vi "find_handle_pose.vi"(7 "Parameters":T1={"Stimulus"={"Type"=enum."Off", "Delay"=0, "Amplitude"=[0.0, 0.0, 0.0], "Injection point"=enum."Total pose", "Closed loop"=FALSE, "Offset"=[0.0, 0.0, 0.0], "Tip -> world"=TRUE}, "Goal Filter A"={"Lower Fc"=0.0, "Lower Q"=0.15, "Scale factor"=0.0, "Upper Fc"=0.0075, "Upper Q"=0.01, "Manip zeroing"=0.001, "Speedup max"=150.0, "Speedup thresh"=5.0, "Speedup nonlin"=3.0, "V limit"=300.0, "V limit range"=300.0}, "Mode controls"={"Hold"=FALSE, "Cancellation"=FALSE, "Goal filter"=FALSE, "Trigger"=FALSE}, "Manipulator type"=enum."Current piezo", "Manipulator calibration"={"Inverse Kinematics"=[[-0.4736411481566654, -0.25724305819165183, -1.1087933259307599], [0.296735958809338, -0.258643951607561, -1.0971603505753995], [-0.043664688535758014, 0.44635679599468125, -1.1035515399424176]], "Handle transform"=[[3.281333089700394, 0.23462731743748497, 0.17832137948371765, -8265.081657965618], [-0.20249098046098263, 2.6933210343964133, -0.2815002765708058, -33565.66155248382], [-0.14581170473284072, 0.6821648518522063, 0.8833544952169589, 26862.18782130476], [-1.1202010727438122e-18, 5.861467994999758e-19, 1.760134464394436e-18, 0.999999999999992]], "Tip offset"=[0.0, 0.0, 36200.0], "Probe calibration"=[], "Pivot position"=[0.0, 0.0, -11360.0], "Axial filter"={"filter structure"=enum."IIR 2nd Order", "Reverse Coefficients"=[0.0, 0.0], "Forward Coefficients"=[1.0, 0.0, 0.0]}, "Lateral filter"={"filter structure"=enum."IIR 2nd Order", "Reverse Coefficients"=[0.0, 0.0], "Forward Coefficients"=[1.0, 0.0, 0.0]}}, "Charge piezo"={"Capacitance"=4e-08, "V min"=-235.0, "V max"=50.0, "- margin"=465.0, "+ margin"=0.001, "I max"=40000.0, "I sat"=90000000.0, "R series"=5.0, "R shunt"=1000.0, "Fault V"=0.0, "Start Fault V"=0.0, "Start Cycles"=0, "Prop gain"=1e-06, "Int gain"=0.0, "Diff gain"=0.0}, "Network"={"Remote Host"="192.168.1.3", "Send Status"=TRUE, "Send Port"=0, "Recv Commands"=FALSE, "Recv Port"=0}, "Goal Filter B"={"Lower Fc"=1.0, "Lower Q"=2.0, "Scale factor"=61557.0, "Upper Fc"=20.0, "Upper Q"=61557.0, "Manip zeroing"=2.0, "Speedup max"=1.0, "Speedup thresh"=300.0, "Speedup nonlin"=3.0, "V limit"=300.0, "V limit range"=300.0}, "Cancellation"={"Bandwidth"=0.0, "Delay"=0, "Stack travel"=0.0, "Saturation pos"=0.0075, "Slew Limit"=0.01, "Turnoff zeroing"=0.001, "Bypass"=FALSE}, "Transition time"=3.0} {"Transition time" format="%_3f"; "Cancellation"."Slew Limit" format="%#_3p"; "Cancellation"."Saturation pos" format="%#.1f"; "Cancellation"."Stack travel" format="%#.1f"; "Cancellation"."Turnoff zeroing" format="%#_6e"; "Cancellation"."Delay" step=1; "Cancellation"."Bandwidth" min=10 max=1000 step=10; "Goal Filter B"."V limit range" format="%_3p"; "Goal Filter B"."V limit" format="%_3p"; "Goal Filter B"."Speedup nonlin" format="%_3p"; "Goal Filter B"."Upper Q" format="%_3f"; "Goal Filter B"."Upper Fc" format="%_3p"; "Goal Filter B"."Lower Q" format="%_3f"; "Goal Filter B"."Speedup thresh" format="%_3p"; "Goal Filter B"."Speedup max" format="%_3p"; "Goal Filter B"."Manip zeroing" format="%_3p"; "Goal Filter B"."Scale factor" format="%_3f"; "Goal Filter B"."Lower Fc" format="%_3p"; "Charge piezo"."I sat" format="%#_6p"; "Charge piezo"."+ margin" format="%#_6p"; "Charge piezo"."- margin" format="%#_6p"; "Charge piezo"."Start Fault V" format="%#_6p"; "Charge piezo"."R shunt" format="%#_6p"; "Charge piezo"."Prop gain" format="%#_6p"; "Charge piezo"."Fault V" format="%#_6p"; "Charge piezo"."I max" format="%#_6p"; "Charge piezo"."Diff gain" format="%#_6p"; "Charge piezo"."Int gain" format="%#_6p"; "Charge piezo"."R series" format="%#_6p"; "Charge piezo"."Capacitance" format="%#_6p"; "Manipulator calibration"."Probe calibration" format="%#.1f"; "Manipulator calibration"."Handle transform" format="%#_3f"; "Manipulator calibration"."Inverse Kinematics" format="%#_3f"; "Goal Filter A"."V limit range" format="%_3p"; "Goal Filter A"."V limit" format="%_3p"; "Goal Filter A"."Speedup nonlin" format="%_3p"; "Goal Filter A"."Upper Q" format="%_3f"; "Goal Filter A"."Upper Fc" format="%_3p"; "Goal Filter A"."Lower Q" format="%_3f"; "Goal Filter A"."Speedup thresh" format="%_3p"; "Goal Filter A"."Speedup max" format="%_3p"; "Goal Filter A"."Manip zeroing" format="%_3p"; "Goal Filter A"."Scale factor" format="%_3f"; "Goal Filter A"."Lower Fc" format="%_3p"; "Stimulus"."Offset" step=100; "Stimulus"."Amplitude" step=100; "Stimulus"."Delay" step=100}, 10 "Zeroing offset":sgl[](array[numeric])) -> (0 "Handle pose":T7 format="%#_5f", 1 "Central tip position":sgl[](array[numeric]), 2 "Manipulator pose":T7 format="%#_5f", 3 "Tip position":sgl[](array[numeric]))   [LabVIEW 2010]
uses:
  <vilib>/Analysis/Matrix/Datatypes/RealMatrix.ctl
  testing/Micron params.ctl
  testing/stimulus.ctl
  testing/injection_point.ctl
  filtering/goal_filter_parms.ctl
  testing/mode_conrols.ctl
  testing/manipulator_cal.ctl
  asap/labview/testing/probe_calibration.ctl
  manipulator/Charge controller params.ctl
  host/network_params.ctl
  cancellation/im_control_params.ctl
  <vilib>/Analysis/Matrix/Numeric/Conversions/Array To Matrix - RA2.vi
  <vilib>/Analysis/baseanly.llb/A x Vector.vi
  <vilib>/Analysis/Matrix/Numeric/Conversions/Array To Matrix - RA.vi
  utilities/labview/norm_vec.vi
  <vilib>/Analysis/Matrix/NI_Matrix.lvlib
  <vilib>/Analysis/NI_AALBase.lvlib
panel:
  in  "Use Raw Data (ignore Kalman Filter)":bool
  # "Offset to apply to central tip position to keep manipulator centered."
  # "Tip position in world coordinates"
  # "Manipulator pose as computed in in the main micron_update loop and stored in the \"Manipulator pose\" shared var."
  # "Intended tip position implied by handle pose."
  # "Pose of the handle.  When the tip is centered, the handle and manipulator pose are identical."
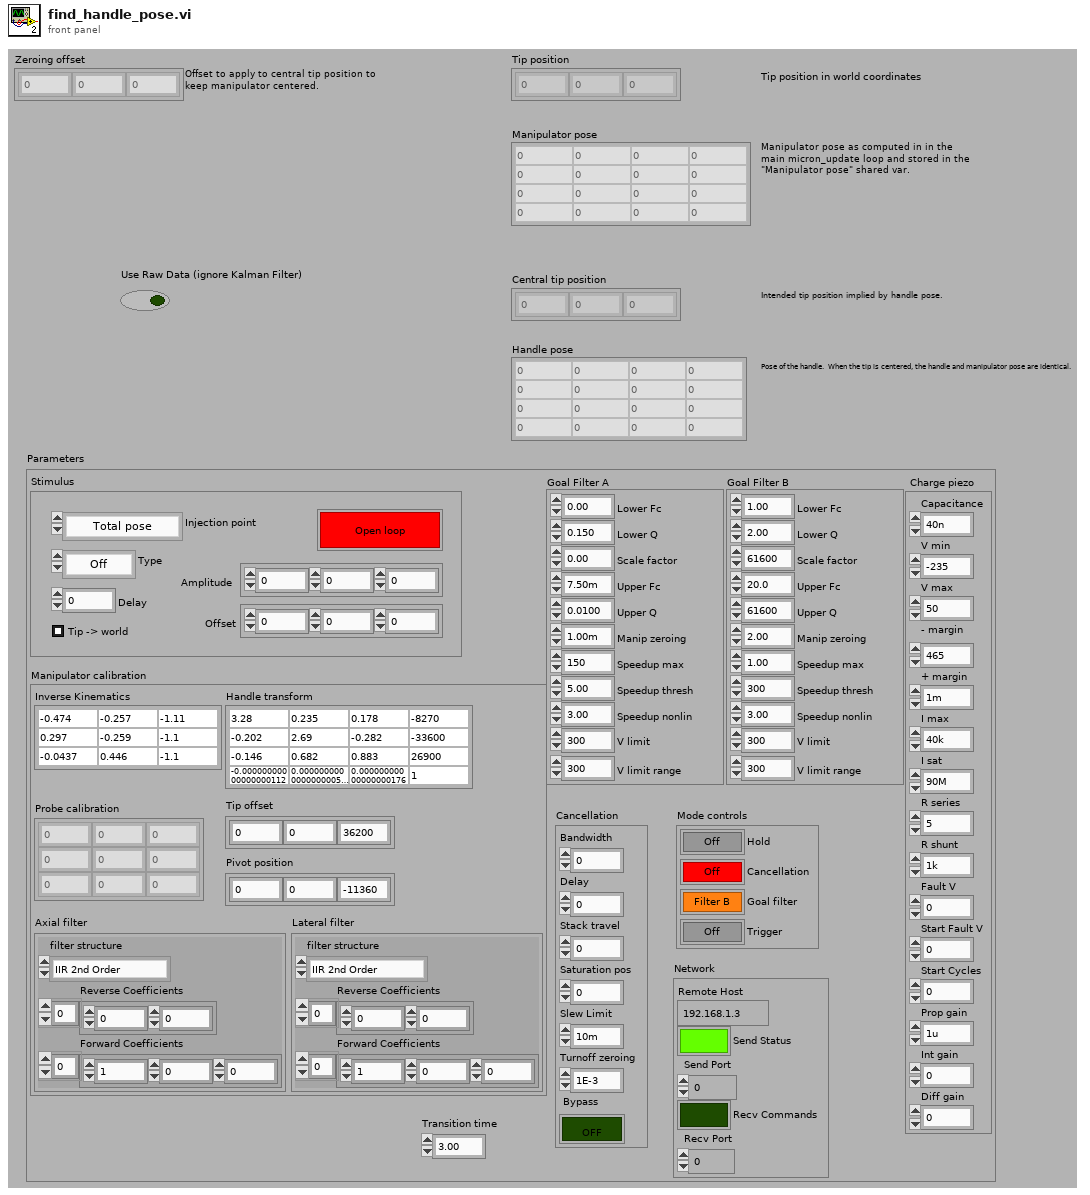
[diagram p1: front panel]
types:
  T1 = typedef "Micron params.ctl" = cluster{"Stimulus":T2, "Goal Filter A":T4, "Mode controls":T5, "Manipulator type":enum16{"Current piezo", "Voltage piezo"}, "Manipulator calibration":T6, "Charge piezo":T9, "Network":T10, "Goal Filter B":T4, "Cancellation":T11, "Transition time":sgl}
  T2 = typedef "stimulus.ctl" = cluster{"Type":enum16{"Off", "Step", "Sine", "Triangle", "Arbitrary"}, "Delay":i32, "Amplitude":sgl[], "Injection point":T3, "Closed loop":bool, "Offset":sgl[], "Tip -> world":bool}
  T3 = typedef "injection_point.ctl" = enum16{"Total pose", "V limiter", "Goal position", "Tip error (manip)", "Inverse kin", "Controller", "Stack position", "Stack drive", "DAC"}
  T4 = typedef "goal_filter_parms.ctl" = cluster{"Lower Fc":sgl, "Lower Q":sgl, "Scale factor":sgl, "Upper Fc":sgl, "Upper Q":sgl, "Manip zeroing":sgl, "Speedup max":sgl, "Speedup thresh":sgl, "Speedup nonlin":sgl, "V limit":sgl, "V limit range":sgl}
  T5 = typedef "mode_conrols.ctl" = cluster{"Hold":bool, "Cancellation":bool, "Goal filter":bool, "Trigger":bool}
  T6 = typedef "manipulator_cal.ctl" = cluster{"Inverse Kinematics":T7, "Handle transform":T7, "Tip offset":sgl[], "Probe calibration":T8, "Pivot position":sgl[], "Axial filter":cluster{"filter structure":enum32{"IIR 2nd Order", "IIR 4th Order"}, "Reverse Coefficients":dbl[], "Forward Coefficients":dbl[]}, "Lateral filter":cluster{"filter structure":enum32{"IIR 2nd Order", "IIR 4th Order"}, "Reverse Coefficients":dbl[], "Forward Coefficients":dbl[]}}
  T7 = typedef "NI_Matrix.lvlib/RealMatrix.ctl" = dbl[][]
  T8 = typedef "probe_calibration.ctl" = sgl[][]
  T9 = typedef "Charge controller params.ctl" = cluster{"Capacitance":sgl, "V min":sgl, "V max":sgl, "- margin":sgl, "+ margin":sgl, "I max":sgl, "I sat":sgl, "R series":sgl, "R shunt":sgl, "Fault V":sgl, "Start Fault V":sgl, "Start Cycles":i32, "Prop gain":sgl, "Int gain":sgl, "Diff gain":sgl}
  T10 = typedef "network_params.ctl" = cluster{"Remote Host":string, "Send Status":bool, "Send Port":u16, "Recv Commands":bool, "Recv Port":u16}
  T11 = typedef "im_control_params.ctl" = cluster{"Bandwidth":sgl, "Delay":i32, "Stack travel":sgl, "Saturation pos":sgl, "Slew Limit":sgl, "Turnoff zeroing":sgl, "Bypass":bool}
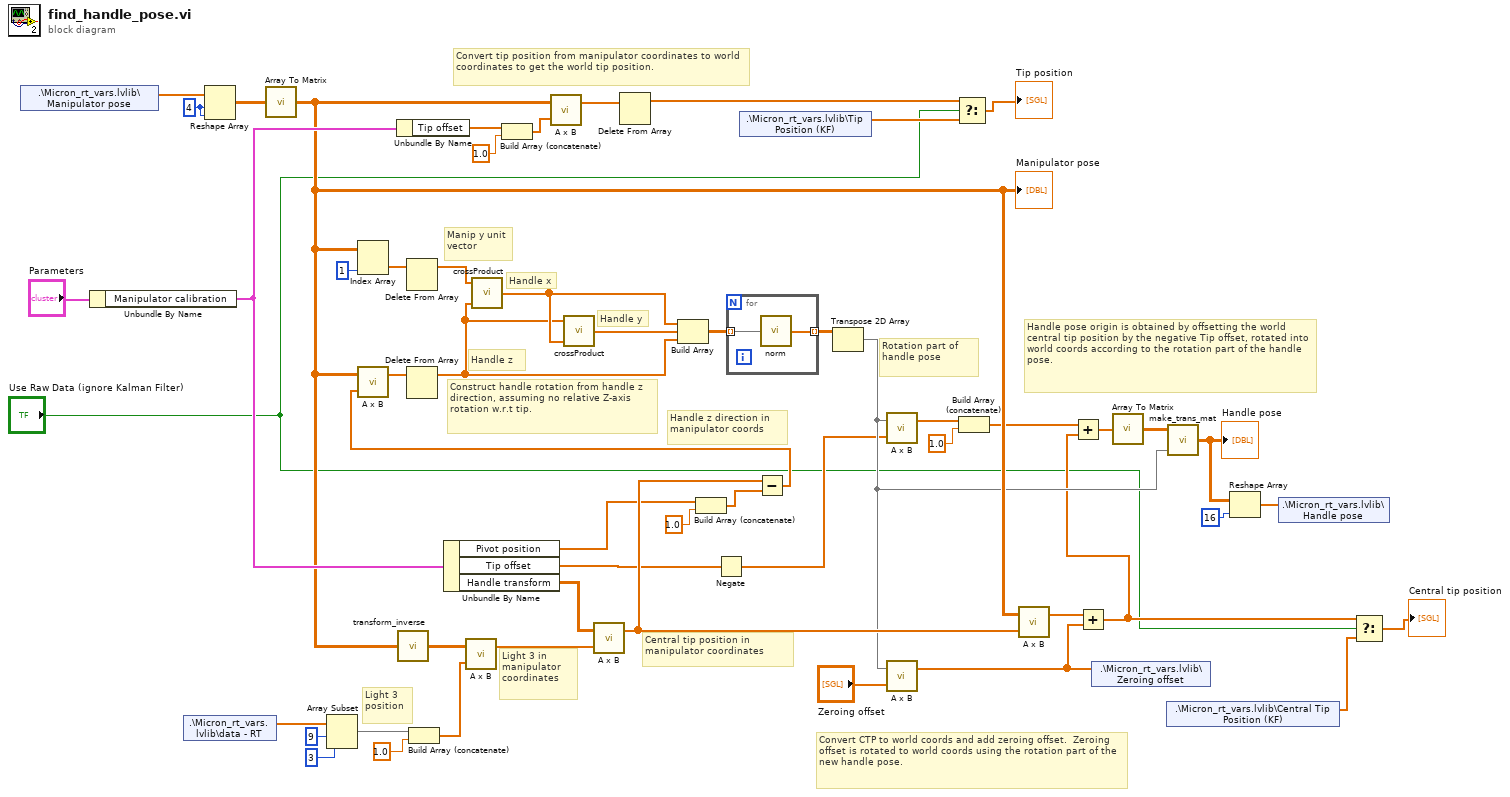
[diagram p0: block diagram]
diagram:
  w54 = 4 ("dimension size")
  # "Handle pose origin is obtained by offsetting the world central tip position by the negative Tip offset, rotated into world coords according to the rotation part of the handle pose."
  # "Convert CTP to world coords and add zeroing offset.  Zeroing offset is rotated to world coords using the rotation part of the new handle pose."
  # "Rotation part of handle pose"
  # "Convert tip position from manipulator coordinates to world coordinates to get the world tip position."
  # "Handle z direction in manipulator coords"
  # "Central tip position in manipulator coordinates"
  # "Light 3 in manipulator  coordinates"
  # "Light 3 position"
  # "Construct handle rotation from handle z direction, assuming no relative Z-axis rotation w.r.t tip."
  # "Handle y"
  # "Handle x"
  # "Handle z"
  # "Manip y unit vector"
  n1 = shared-variable ".\\Micron_rt_vars.lvlib\\Manipulator pose"() -> (w53:sgl[])  [unwired: 2 out]
  n2 = Unbundle By Name("Parameters") -> ("Manipulator calibration"=w23:T6)
  n3 = shared-variable ".\\Micron_rt_vars.lvlib\\data - RT"() -> (w52:sgl[])  [unwired: 2 out]
  n4 = Reshape Array(w53, w54, w54) -> (w32:sgl[][])
  n5 = call-poly <vilib>:"Array To Matrix.vi"("Real 2D Array"=w32) -> ("Real Matrix"=w22:T7)
  "Manipulator pose" <- w22
  n6 = Array Subset(array=w52, index=9, length=3) -> (w38:sgl[])
  n7 = Index Array(array=w22, index (col)=1 ("disabled index (col)")) -> (element=w49:dbl[])  [unwired: 1 in]
  n8 = Unbundle By Name(w23) -> ("Tip offset"=w26:sgl[])
  n9 = call "transform_inverse.vi"("Transform"=w22) -> ("Inverse transform"=w40:T7)
  n10 = Delete From Array(array=w49) -> (array with subset deleted=w46:dbl[])  [unwired: 2 in, 1 out]
  n11 = Build Array (concatenate)(w38, sgl 1.0) -> (w37:sgl[])
  n12 = Unbundle By Name(w23) -> ("Pivot position"=w25:sgl[], "Tip offset"=w13:sgl[], "Handle transform"=w24:T7)
  n13 = call-poly <vilib>:"A x B.vi"("Vector"=w37, "A"=w40) -> ("A x Vector"=w36:dbl[])  [unwired: 1 out]
  n14 = Build Array (concatenate)(w26, sgl 1.0 ("Numeric")) -> (w29:sgl[])
  n15 = call-poly <vilib>:"A x B.vi"("Vector"=w29, "A"=w22) -> ("A x Vector"=w31:dbl[])  [unwired: 1 out]
  n16 = call-poly <vilib>:"A x B.vi"("Vector"=w36, "A"=w24) -> ("A x Vector"=w33:dbl[])  [unwired: 1 out]
  n17 = Delete From Array(array=w31) -> (array with subset deleted=w7:dbl[])  [unwired: 2 in, 1 out]
  n18 = Build Array (concatenate)(w25, sgl 1.0 ("Numeric")) -> (w21:sgl[])
  n19 = Negate(x=w13) -> (-x=w12:sgl[])
  n20 = shared-variable ".\\Micron_rt_vars.lvlib\\Tip Position (KF)"() -> (w5:sgl[])  [unwired: 2 out]
  n21 = Subtract(x=w33, y=w21) -> (x-y=w34:dbl[])
  n22 = call-poly <vilib>:"A x B.vi"("Vector"=w34, "A"=w22) -> ("A x Vector"=w47:dbl[])  [unwired: 1 out]
  n23 = Delete From Array(array=w47) -> (array with subset deleted=w43:dbl[])  [unwired: 2 in, 1 out]
  n24 = call "crossProduct.vi"("B"=w43, "A"=w46) -> ("A x B"=w45:dbl[])  [unwired: 3 out]
  n25 = call "crossProduct.vi"("B"=w45, "A"=w43) -> ("A x B"=w44:dbl[])  [unwired: 3 out]
  n26 = Build Array(w45, w44, w43) -> (w42:dbl[][])
  n27 = for {
    tunnel: w42 -> [w56] mode=indexing
    tunnel: [w55] -> w41 mode=indexing
    n28 = call-poly "norm.vi"("vector"=w56) -> ("normalized vector"=w55:dbl[])  [unwired: 4 out]
  }
  n29 = Transpose 2D Array(2D array=w41) -> (transposed array=w14:dbl[][])
  n30 = call-poly <vilib>:"A x B.vi"("Vector"=w12, "A"=w14) -> ("A x Vector"=w10:dbl[])  [unwired: 1 out]
  n31 = call-poly <vilib>:"A x B.vi"("Vector"="Zeroing offset", "A"=w14) -> ("A x Vector"=w18:dbl[])  [unwired: 1 out]
  n32 = Select(t=w7, s="Use Raw Data (ignore Kalman Filter)", f=w5) -> (s? t:f=→"Tip position":dbl[])
  n33 = Build Array (concatenate)(w10, sgl 1.0 ("Numeric")) -> (w9:dbl[])
  n34 = call-poly <vilib>:"A x B.vi"("Vector"=w33, "A"=w22) -> ("A x Vector"=w20:dbl[])  [unwired: 1 out]
  n35 = Add(x=w20, y=w18) -> (x+y=w4:dbl[])
  n36 = Add(x=w9, y=w4) -> (x+y=w8:dbl[])
  n37 = shared-variable ".\\Micron_rt_vars.lvlib\\Zeroing offset"(w18) -> ()  [unwired: 2 out]
  n38 = call-poly <vilib>:"Array To Matrix.vi"("Real 1D Array"=w8) -> ("Real Matrix (Column Vector)"=w35:T7)
  n39 = shared-variable ".\\Micron_rt_vars.lvlib\\Central Tip Position (KF)"() -> (w3:sgl[])  [unwired: 2 out]
  n40 = call "make_trans_mat.vi"("Rotation"=w14, "Translation"=w35) -> ("Result"=w15:T7)  [unwired: 3 out]
  "Handle pose" <- w15
  n41 = Reshape Array(w15, 16 ("dimension size")) -> (w17:dbl[])
  n42 = shared-variable ".\\Micron_rt_vars.lvlib\\Handle pose"(w17) -> ()  [unwired: 2 out]
  n43 = Select(t=w4, s="Use Raw Data (ignore Kalman Filter)", f=w3) -> (s? t:f=→"Central tip position":dbl[])
